vi "Teleop.vi"(10 "Match Info":T1={"Autonomous Elapsed Seconds"=0.0, "TeleOp Elapsed Seconds"=0.0, "Disabled Elapsed Seconds"=0.0, "Visited Autonomous"=FALSE, "Visited TeleOp"=FALSE, "Visited Disabled"=FALSE, "Autonomous Settings"={"Autonomous Style"=enum."Independent", "VI Refnum"=refnum}}, 11 "Call Context":T2) -> ()   [LabVIEW 2019]
doc: "This VI is called for each TeleOp packet received from the DS where the robot is not disabled. It is often used to read from the joysticks and update I/O or to update setpoints for timed control loops. It should complete and return within 20 milliseconds or it may miss DS packets."
uses:
  <vilib>/Rock Robotics/WPI/DriverStation/WPI_DriverStationDerivedRobotMode.ctl
  <vilib>/Rock Robotics/WPI/DriverStation/WPI_DriverStationMatch Info.ctl
  Robot Global Data.vi
  <vilib>/Rock Robotics/WPI/Utilities/WPI_GetSetVariantRefNum.vi
  <vilib>/Rock Robotics/Network Tables/NT Read Number.vi
  <vilib>/Rock Robotics/Network Tables/NT Write Number.vi
panel:
  # "Click here to set min"
  # "Click here to set max"
  # "Click here to set min"
  # "Click here to set max"
  # "Click here to set min"
  # "Click here to set max"
  # "Click here to set min"
  # "Click here to set max"
  # "Click here to set min"
  # "Click here to set max"
  # "Click here to set min"
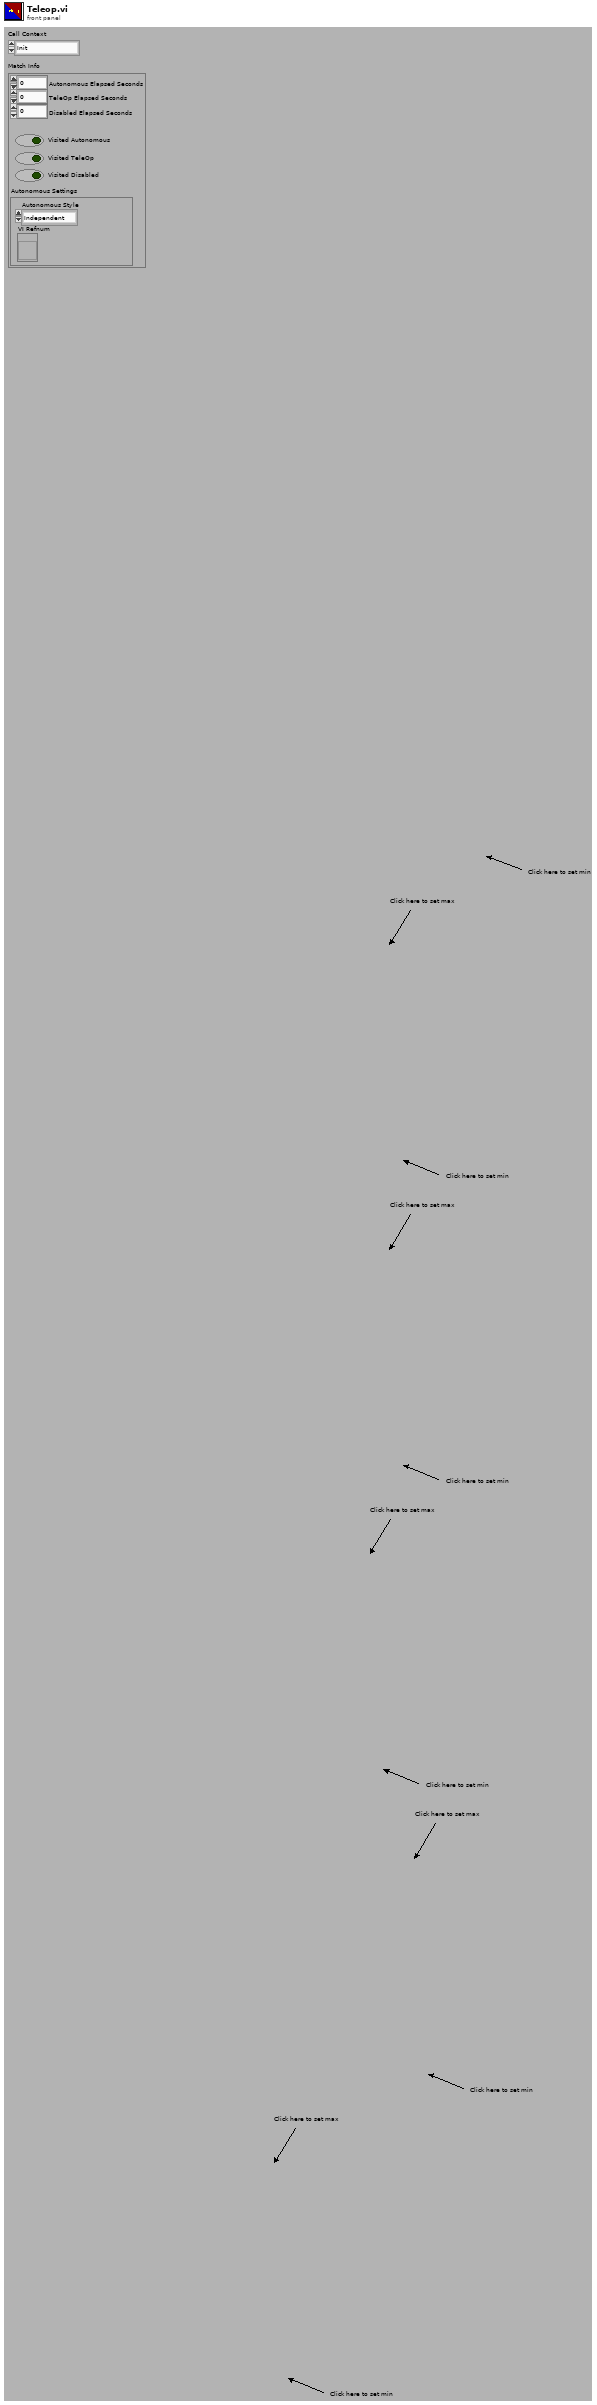
[diagram p1: front panel]
types:
  T1 = typedef "WPI_DriverStationMatch Info.ctl" = cluster{"Autonomous Elapsed Seconds":dbl, "TeleOp Elapsed Seconds":dbl, "Disabled Elapsed Seconds":dbl, "Visited Autonomous":bool, "Visited TeleOp":bool, "Visited Disabled":bool, "Autonomous Settings":cluster{"Autonomous Style":enum16{"Iterative", "Independent"}, "VI Refnum":refnum<vi>}}
  T2 = typedef "WPI_DriverStationDerivedRobotMode.ctl" = enum16{"Init", "Execute", "Stop"}
  T3 = typedef "WPI_MotorControlDeviceRef.ctl" = cluster{"DeviceStatus":errorcluster, "Type":T4, "PWM":cluster{"PWM Channel":T5, "DeadBand":T6}, "CAN":cluster{"Device Number":u8, "SetOutput VI Ref":variant, "GetOutput VI Ref":variant, "Enable VI Ref":variant, "Disable VI Ref":variant, "Data":variant}, "Invert":bool, "DIO PWM":cluster{"PWM \"Enable\" Channel":T5, "DIOChannel":T7, "PWM Rate":dbl}}
  T4 = typedef "WPI_MotorControlType.ctl" = enum16{"PWM", "CAN", "DIO PWM"}
  T5 = typedef "FPGA_DIOPWMChannel.ctl" = enum8{"PWM 0", "PWM 1", "PWM 2", "PWM 3", "PWM 4", "PWM 5", "PWM 6", "PWM 7", "PWM 8", "PWM 9", "PWM MXP 0", "PWM MXP 1", "PWM MXP 2", "PWM MXP 3", "PWM MXP 4", "PWM MXP 5", "PWM MXP 6", "PWM MXP 7", "PWM MXP 8", "PWM MXP 9", "Invalid"}
  T6 = typedef "WPI_PWMDeadband.ctl" = cluster{"Name":string, "maxPositivePwm":i32, "minPositivePwm":i32, "centerPwm":i32, "maxNegativePwm":i32, "minNegativePwm":i32, "angularRange":u16}
  T7 = typedef "FPGA_DIOChannel.ctl" = enum8{"DIO 0", "DIO 1", "DIO 2", "DIO 3", "DIO 4", "DIO 5", "DIO 6", "DIO 7", "DIO 8", "DIO 9", "DIO MXP 0", "DIO MXP 1", "DIO MXP 2", "DIO MXP 3", "DIO MXP 4", "DIO MXP 5", "DIO MXP 6", "DIO MXP 7", "DIO MXP 8", "DIO MXP 9", "DIO MXP 10", "DIO MXP 11", "DIO MXP 12", "DIO MXP 13", "DIO MXP 14", "DIO MXP 15", "SPI Port CS1", "SPI Port CS2", "SPI Port CS3", "SPI Port MISO", "SPI Port MOSI", "Invalid"}
  T8 = typedef "WPI_ServoDeviceRef.ctl" = cluster{"DeviceStatus":errorcluster, "PWM Channel":T5, "DeadBand":T6}
  T9 = typedef "WPI_JoystickDevRef.ctl" = cluster{"Device":T10}
  T10 = typedef "WPI_JoystickDeviceEnum.ctl" = enum16{"USB 0", "USB 1", "USB 2", "USB 3", "USB 4", "USB 5"}
  T11 = typedef "WPI_RobotDriveDevRef.ctl" = cluster{"DevStatus":errorcluster, "Motors[]":T3[], "Square Inputs":bool, "Max Output":dbl}
  T12 = cluster{"JoystickDevRef":T9, "RobotDriveDevRef":T11}
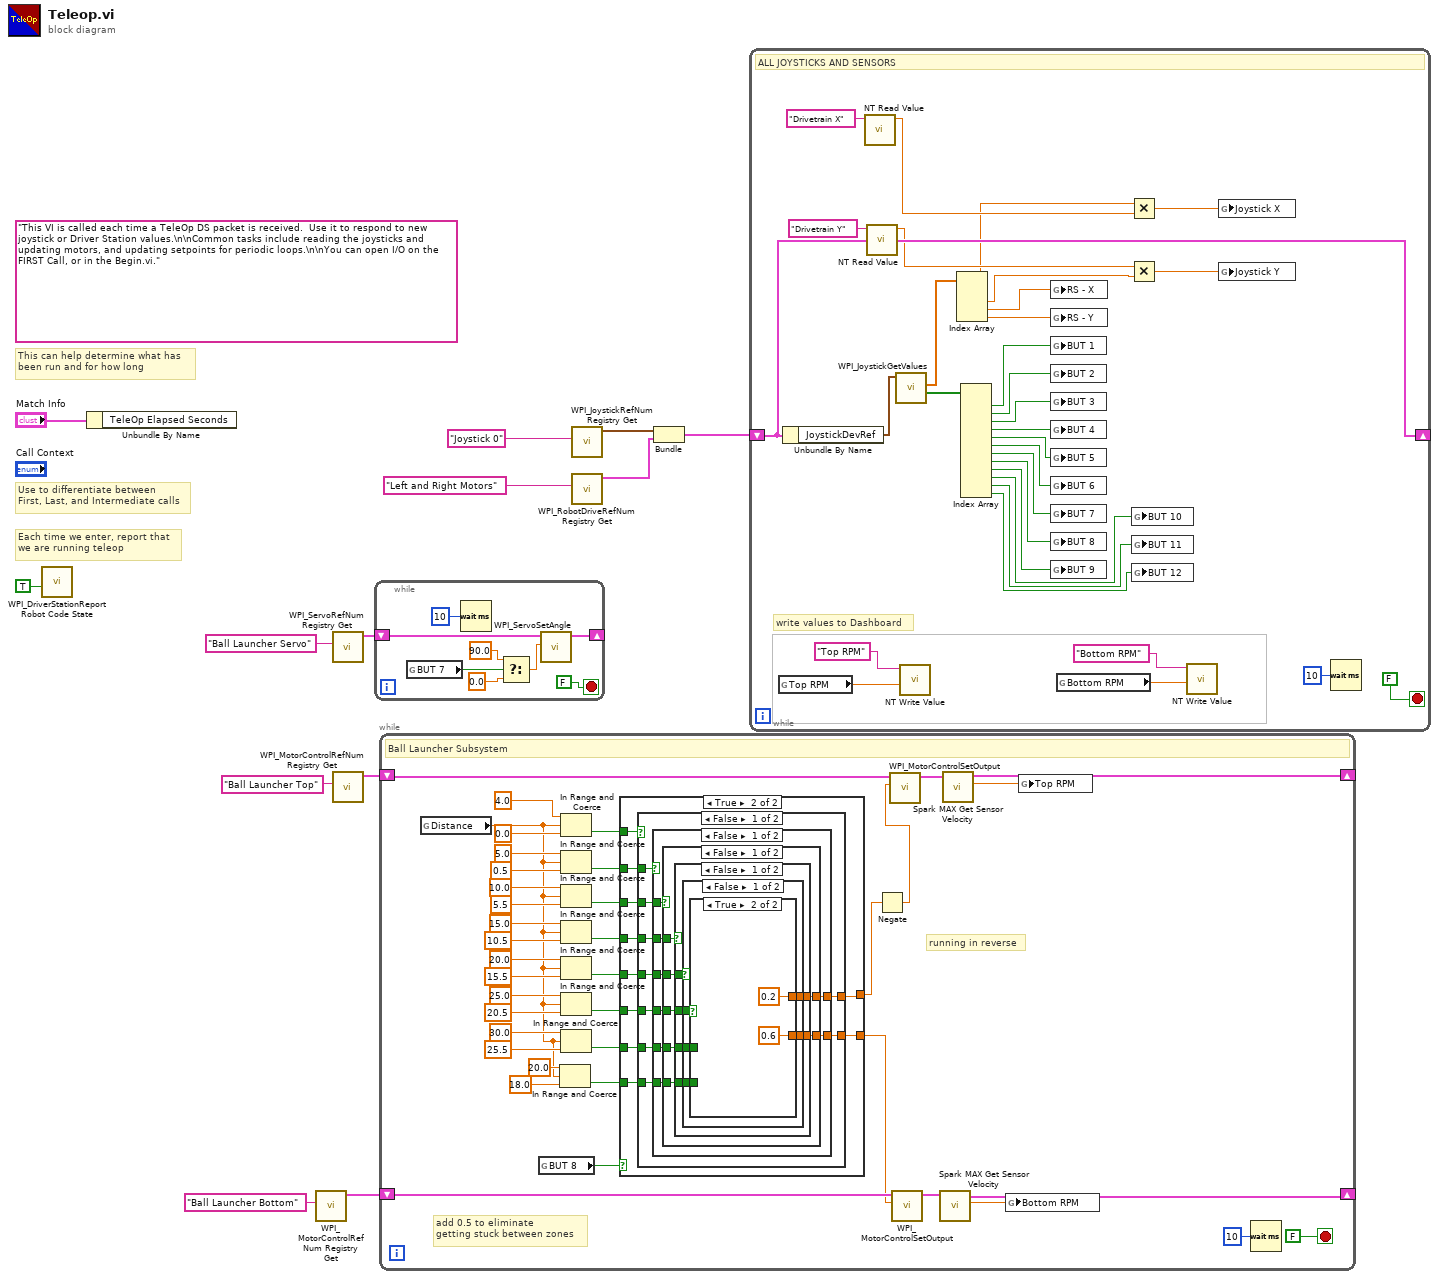
[diagram p0: block diagram]
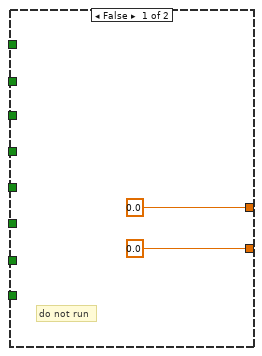
[diagram p2: hidden frame]
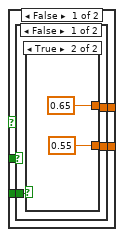
[diagram p3: hidden frame]
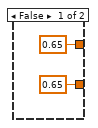
[diagram p4: hidden frame]
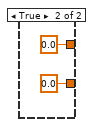
[diagram p5: hidden frame]
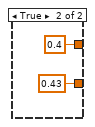
[diagram p6: hidden frame]
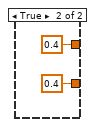
[diagram p7: hidden frame]
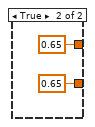
[diagram p8: hidden frame]
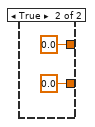
[diagram p9: hidden frame]
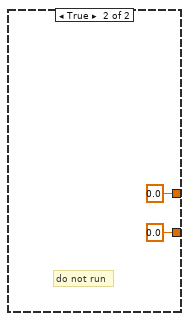
[diagram p10: hidden frame]
diagram:
  (unwired) "This VI is called each time a TeleOp DS packet is received.  Use it to respond to new joystick or Driver Station values.\n\nCommon tasks include reading the joysticks and updating motors, and updating setpoints for periodic loops.\n\nYou can open I/O on the FIRST Call, or in the Begin.vi."
  # "Each time we enter, report that\nwe are running teleop"
  # "Use to differentiate between\nFirst, Last, and Intermediate calls"
  # "This can help determine what has\nbeen run and for how long"
  n1 = call <vilib>:"WPI_DriverStationReport Robot Code State.vi"("TeleOp"=TRUE ("Autonomous")) -> ()  [unwired: 10 in, 1 out]
  n2 = Unbundle By Name("Match Info") -> ()  [unwired: 1 out]
  n3 = call <vilib>:"WPI_MotorControlRefNum Registry Get.vi"("refnum name"="Ball Launcher Bottom") -> ("MotorControlDevRef"=w2:T3)  [unwired: 9 in, 1 out]
  n4 = call <vilib>:"WPI_ServoRefNum Registry Get.vi"("refnum name"="Ball Launcher Servo") -> ("ServoDeviceRef"=w11:T8)  [unwired: 9 in, 1 out]
  n5 = call <vilib>:"WPI_MotorControlRefNum Registry Get.vi"("refnum name"="Ball Launcher Top") -> ("MotorControlDevRef"=w1:T3)  [unwired: 9 in, 1 out]
  n6 = while {
    shift-right: [w17] -> _
    shift-left: w11 -> [w16]
    stop <- FALSE stop-if-true
    n7 = global read "Robot Global Data.vi" "BUT 7"() -> (w14:bool)
    n8 = Wait (ms)(milliseconds to wait=u32 10) -> ()  [unwired: 1 out]
    n9 = Select(t=90.0, s=w14, f=0.0) -> (s? t:f=w15:dbl)
    n10 = call <vilib>:"WPI_ServoSetAngle.vi"("Angle"=w15, "ServoDeviceRef"=w16) -> ("ServoDeviceRef"=w17:T8)  [unwired: 8 in, 1 out]
  }
  n11 = while {
    shift-right: [w57] -> _
    shift-left: w1 -> [w53]
    shift-right: [w58] -> _
    shift-left: w2 -> [w51]
    stop <- FALSE stop-if-true
    # "running in reverse"
    # "add 0.5 to eliminate\ngetting stuck between zones"
    # "Ball Launcher Subsystem"
    n12 = global read "Robot Global Data.vi" "Distance"() -> (w22:dbl)
    n13 = global read "Robot Global Data.vi" "BUT 8"() -> (w50:bool)
    n14 = In Range and Coerce(upper limit=20.0, x=w22, lower limit=18.0) -> (In Range?=w25:bool)  [unwired: 1 out]
    n15 = In Range and Coerce(upper limit=4.0, x=w22, lower limit=0.0) -> (In Range?=w28:bool)  [unwired: 1 out]
    n16 = In Range and Coerce(upper limit=5.0, x=w22, lower limit=0.5) -> (In Range?=w29:bool)  [unwired: 1 out]
    n17 = In Range and Coerce(upper limit=10.0, x=w22, lower limit=5.5) -> (In Range?=w48:bool)  [unwired: 1 out]
    n18 = In Range and Coerce(upper limit=15.0, x=w22, lower limit=10.5) -> (In Range?=w47:bool)  [unwired: 1 out]
    n19 = In Range and Coerce(upper limit=20.0, x=w22, lower limit=15.5) -> (In Range?=w46:bool)  [unwired: 1 out]
    n20 = In Range and Coerce(upper limit=25.0, x=w22, lower limit=20.5) -> (In Range?=w45:bool)  [unwired: 1 out]
    n21 = In Range and Coerce(upper limit=30.0, x=w22, lower limit=25.5) -> (In Range?=w44:bool)  [unwired: 1 out]
    n22 = case shown="True" w50 {
      tunnel: [0.0 ("Output") w65] -> w26
      tunnel: [0.0 ("Output") w64] -> w49
      tunnel: w28 -> [_ w72]
      tunnel: w48 -> [_ w70]
      tunnel: w47 -> [_ w69]
      tunnel: w46 -> [_ w68]
      tunnel: w45 -> [_ w67]
      tunnel: w44 -> [_ w66]
      tunnel: w29 -> [_ w71]
      tunnel: w25 -> [_ w63]
      frame False {
        # "do not run"
      }
      frame True {
        n23 = case shown="False" w72 {
          tunnel: w71 -> [w81 _]
          tunnel: w70 -> [w80 _]
          tunnel: w69 -> [w79 _]
          tunnel: w68 -> [w78 _]
          tunnel: w67 -> [w77 _]
          tunnel: w66 -> [w76 _]
          tunnel: [w75 0.0 ("Output")] -> w65
          tunnel: [w74 0.0 ("Output")] -> w64
          tunnel: w63 -> [w73 _]
          frame False {
            n24 = case shown="False" w81 {
              tunnel: w80 -> [w89 _]
              tunnel: w79 -> [w88 _]
              tunnel: w78 -> [w87 _]
              tunnel: w77 -> [w86 _]
              tunnel: w76 -> [w85 _]
              tunnel: [w84 0.0 ("Output")] -> w75
              tunnel: [w83 0.0 ("Output")] -> w74
              tunnel: w73 -> [w82 _]
              frame False {
                n25 = case shown="False" w89 {
                  tunnel: w88 -> [w96 _]
                  tunnel: w87 -> [w95 _]
                  tunnel: w86 -> [w94 _]
                  tunnel: w85 -> [w93 _]
                  tunnel: [w92 0.65 ("Output")] -> w84
                  tunnel: [w91 0.65 ("Output")] -> w83
                  tunnel: w82 -> [w90 _]
                  frame False {
                    n26 = case shown="False" w96 {
                      tunnel: w95 -> [w102 _]
                      tunnel: w94 -> [w101 _]
                      tunnel: w93 -> [w100 _]
                      tunnel: [w99 0.4 ("Output")] -> w92
                      tunnel: [w98 0.4 ("Output")] -> w91
                      tunnel: w90 -> [w97 _]
                      frame False {
                        n27 = case shown="False" w102 {
                          tunnel: w101 -> [w107 _]
                          tunnel: w100 -> [w106 _]
                          tunnel: [w105 0.4 ("Output")] -> w99
                          tunnel: [w104 0.43 ("Output")] -> w98
                          tunnel: w97 -> [w103 _]
                          frame False {
                            n28 = case shown="True" w107 {
                              tunnel: w106 -> [w111 _]
                              tunnel: [w110 0.2 ("Output")] -> w105
                              tunnel: [w109 0.6 ("Output")] -> w104
                              tunnel: w103 -> [w108 _]
                              frame False {
                                n29 = case shown="False" w111 {
                                tunnel: [w113 0.0 ("Output")] -> w110
                                tunnel: [w112 0.0 ("Output")] -> w109
                                tunnel: w108 -> [w114 _]
                                frame False {
                                n30 = case shown="True" w114 {
                                tunnel: [0.65 ("Output") 0.65 ("Output")] -> w113
                                tunnel: [0.65 ("Output") 0.55 ("Output")] -> w112
                                frame False {
                                }
                                frame True {
                                }
                                }
                                }
                                frame True {
                                }
                                }
                              }
                              frame True {
                              }
                            }
                          }
                          frame True {
                          }
                        }
                      }
                      frame True {
                      }
                    }
                  }
                  frame True {
                  }
                }
              }
              frame True {
              }
            }
          }
          frame True {
            # "do not run"
          }
        }
      }
    }
    n31 = Negate(x=w26) -> (-x=w27:dbl)
    n32 = call <vilib>:"WPI_MotorControlSetOutput.vi"("Output"=w27, "MotorControlDevRef"=w53) -> ("MotorControlDevRef"=w54:T3)  [unwired: 7 in, 2 out]
    n33 = call <vilib>:"WPI_MotorControlSetOutput.vi"("Output"=w49, "MotorControlDevRef"=w51) -> ("MotorControlDevRef"=w52:T3)  [unwired: 7 in, 2 out]
    n34 = call <vilib>:"Spark MAX Get Sensor Velocity.vi"("MotorControlDevRef in"=w52) -> ("Sensor Velocity"=w55:dbl, "MotorControlDevRef out"=w58:T3)  [unwired: 7 in, 2 out]
    n35 = call <vilib>:"Spark MAX Get Sensor Velocity.vi"("MotorControlDevRef in"=w54) -> ("Sensor Velocity"=w56:dbl, "MotorControlDevRef out"=w57:T3)  [unwired: 7 in, 2 out]
    n36 = global write "Robot Global Data.vi" "Bottom RPM"(w55) -> ()
    n37 = global write "Robot Global Data.vi" "Top RPM"(w56) -> ()
    n38 = Wait (ms)(milliseconds to wait=u32 10) -> ()  [unwired: 1 out]
  }
  n39 = call <vilib>:"WPI_JoystickRefNum Registry Get.vi"("refnum name"="Joystick 0") -> ("JoystickDevRef"=w5:T9)  [unwired: 1 in, 9 out]
  n40 = call <vilib>:"WPI_RobotDriveRefNum Registry Get.vi"("refnum name"="Left and Right Motors") -> ("RobotDriveDevRef"=w4:T11)  [unwired: 1 in, 9 out]
  n41 = Bundle("JoystickDevRef"=w5, "RobotDriveDevRef"=w4) -> (w3:T12)  [unwired: 1 out]
  n42 = while {
    shift-right: [w149] -> _
    shift-left: w3 -> [w149]
    stop <- FALSE stop-if-true
    # "write values to Dashboard"
    # "ALL JOYSTICKS AND SENSORS"
    n43 = global read "Robot Global Data.vi" "Top RPM"() -> (w143:dbl)
    n44 = Unbundle By Name(w149) -> ("JoystickDevRef"=w163:T9)
    n45 = call-poly <vilib>:"NT Read Value.vi"("Name"="Drivetrain X") -> ("Numeric"=w137:dbl)  [unwired: 9 in, 1 out]
    n46 = call-poly <vilib>:"NT Read Value.vi"("Name"="Drivetrain Y") -> ("Numeric"=w138:dbl)  [unwired: 9 in, 1 out]
    n47 = call <vilib>:"WPI_JoystickGetValues.vi"("JoystickDevRef"=w163) -> ("Buttons"=w162:bool[], "Axes"=w148:dbl[])  [unwired: 6 in, 3 out]
    n48 = call-poly <vilib>:"NT Write Value.vi"("Numeric"=w143, "Name"="Top RPM") -> ()  [unwired: 9 in, 1 out]
    n49 = Index Array(array=w148) -> (element #1=w134:dbl, element #2=w133:dbl, element #3=w135:dbl, element #4=w146:dbl)  [unwired: 4 in]
    n50 = Index Array(array=w162) -> (element #1=w161:bool, element #2=w160:bool, element #3=w159:bool, element #4=w158:bool, element #5=w157:bool, element #6=w156:bool, element #7=w155:bool, element #8=w154:bool, element #9=w153:bool, element #10=w152:bool, element #11=w151:bool, element #12=w150:bool)  [unwired: 12 in]
    n51 = global write "Robot Global Data.vi" "RS - X"(w135) -> ()
    n52 = global write "Robot Global Data.vi" "RS - Y"(w146) -> ()
    n53 = global write "Robot Global Data.vi" "BUT 1"(w161) -> ()
    n54 = global write "Robot Global Data.vi" "BUT 2"(w160) -> ()
    n55 = global write "Robot Global Data.vi" "BUT 3"(w159) -> ()
    n56 = global write "Robot Global Data.vi" "BUT 4"(w158) -> ()
    n57 = global write "Robot Global Data.vi" "BUT 5"(w157) -> ()
    n58 = global write "Robot Global Data.vi" "BUT 6"(w156) -> ()
    n59 = global write "Robot Global Data.vi" "BUT 7"(w155) -> ()
    n60 = global write "Robot Global Data.vi" "BUT 8"(w154) -> ()
    n61 = global write "Robot Global Data.vi" "BUT 9"(w153) -> ()
    n62 = global read "Robot Global Data.vi" "Bottom RPM"() -> (w141:dbl)
    n63 = Multiply(x=w134, y=w137) -> (x*y=w136:dbl)
    n64 = Multiply(x=w138, y=w133) -> (x*y=w147:dbl)
    n65 = global write "Robot Global Data.vi" "BUT 10"(w152) -> ()
    n66 = global write "Robot Global Data.vi" "BUT 11"(w151) -> ()
    n67 = global write "Robot Global Data.vi" "BUT 12"(w150) -> ()
    n68 = call-poly <vilib>:"NT Write Value.vi"("Numeric"=w141, "Name"="Bottom RPM") -> ()  [unwired: 9 in, 1 out]
    n69 = global write "Robot Global Data.vi" "Joystick X"(w136) -> ()
    n70 = global write "Robot Global Data.vi" "Joystick Y"(w147) -> ()
    n71 = Wait (ms)(milliseconds to wait=u32 10) -> ()  [unwired: 1 out]
  }
